vi "Build_Asylum_SetPISLoop.vi"(6 "outChannelString":string, 7 "whichLoop":i32, 8 "error in (no error)":errorcluster, 9 "PIS Controls":T1, 10 "inChannelString":string, 11 "eventString":string) -> (0 "error out":errorcluster, 3 "Command":string)   [LabVIEW 2016]
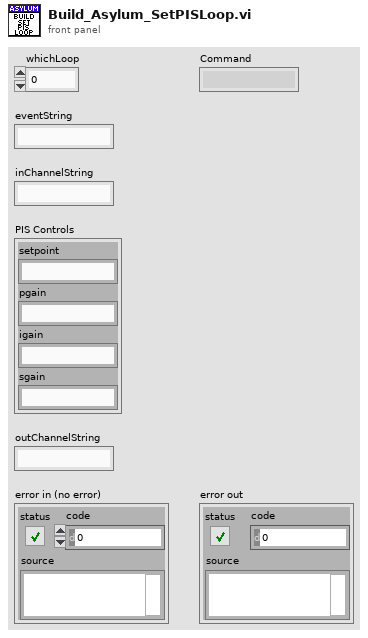
[diagram p1: front panel]
types:
  T1 = cluster{"setpoint":string, "pgain":string, "igain":string, "sgain":string}
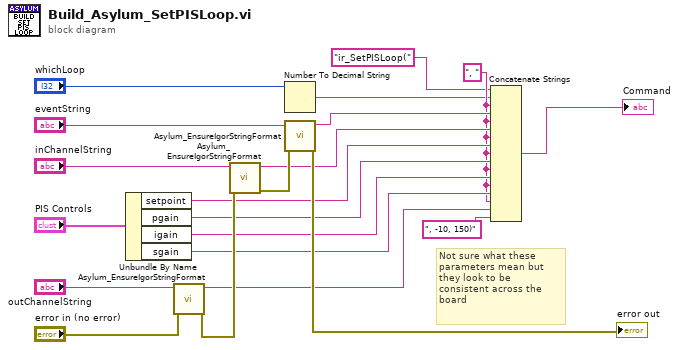
[diagram p0: block diagram]
diagram:
  w8 = ", " ("string")
  # "Not sure what these parameters mean but they look to be consistent across the board"
  n1 = Unbundle By Name("PIS Controls") -> ("setpoint"=w13:string, "pgain"=w14:string, "igain"=w15:string, "sgain"=w16:string)
  n2 = call "Asylum_EnsureIgorStringFormat.vi"("error in (no error)"="error in (no error)", "Value"="outChannelString") -> ("error out"=w21:errorcluster, "Value"=w17:string)  [unwired: 8 in]
  n3 = call "Asylum_EnsureIgorStringFormat.vi"("error in (no error)"=w21, "Value"="inChannelString") -> ("error out"=w19:errorcluster, "Value"=w12:string)  [unwired: 8 in]
  n4 = Number To Decimal String(number="whichLoop") -> (decimal integer string=w4:string)  [unwired: 1 in]
  n5 = call "Asylum_EnsureIgorStringFormat.vi"("error in (no error)"=w19, "Value"="eventString") -> ("error out"=→"error out":errorcluster, "Value"=w11:string)  [unwired: 8 in]
  n6 = Concatenate Strings("ir_SetPISLoop(" ("string"), w4, w8, w11, w8, w12, w8, w13, w8, w14, w8, w15, w8, w16, w8, w17, ", -10, 150)" ("string")) -> (→"Command":string)
